vi "Update_STS_ZSpec_Param_SubVI.vi"(4 "ZSpec Param List #5":u16, 5 "Boolean":bool, 6 "STS Param List #5":u16, 7 "reference in":refnum<vi>, 8 "reference 4":refnum<vi>, 9 "reference 3":refnum<vi>, 10 "Experiment 6":T1, 11 "Path in":refnum<vi>) -> (3 "Experiment 5":T1)   [LabVIEW 2014]
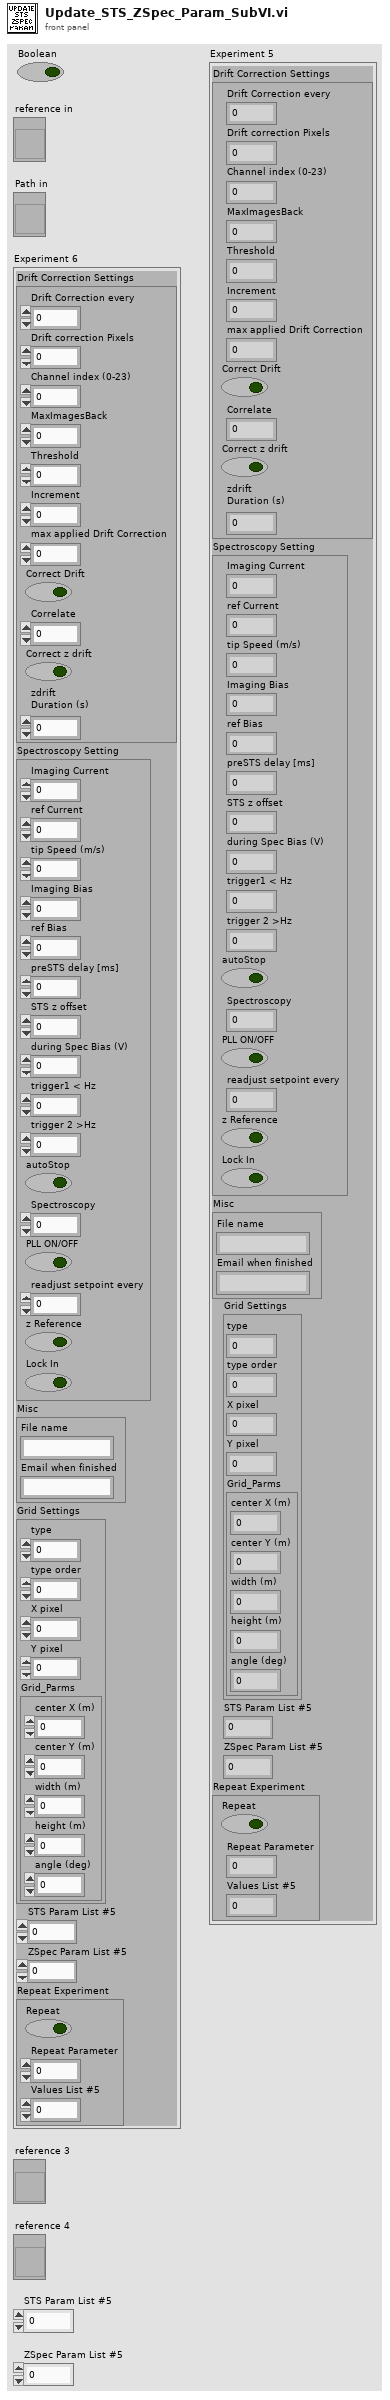
[diagram p1: front panel]
types:
  T1 = cluster{"Drift Correction Settings":cluster{"Drift Correction every":i32, "Drift correction Pixels":i32, "Channel index (0-23)":u8, "MaxImagesBack":i32, "Threshold":i32, "Increment":i32, "max applied Drift Correction":i32, "Correct Drift":bool, "Correlate":u16, "Correct z drift":bool, "zdrift \nDuration (s)":dbl}, "Spectroscopy Setting":cluster{"Imaging Current":dbl, "ref Current":dbl, "tip Speed (m/s)":sgl, "Imaging Bias":dbl, "ref Bias":dbl, "preSTS delay [ms]":u32, "STS z offset":dbl, "during Spec Bias (V)":sgl, "trigger1 < Hz":sgl, "trigger 2 >Hz":sgl, "autoStop":bool, "Spectroscopy":u16, "PLL ON/OFF":bool, "readjust setpoint every ":i32, "z Reference":bool, "Lock In":bool}, "Misc":cluster{"File name":string, "Email when finished":string}, "Grid Settings":cluster{"type":u16, "type order":u16, "X pixel":i32, "Y pixel":i32, "Grid_Parms":cluster{"center X (m)":sgl, "center Y (m)":sgl, "width (m)":sgl, "height (m)":sgl, "angle (deg)":sgl}}, "STS Param List #5 ":u16, "ZSpec Param List #5  ":u16, "Repeat Experiment":cluster{"Repeat":bool, "Repeat Parameter":u16, "Values List #5":i32}}
  T2 = cluster{"Amplitude (mod. signal unit)":sgl, "Lockin on/off status":bool, "Backward sweep":bool, "Number of points":i32, "Channels":string[], "Parameters":string[], "Fixed parameters":string[], "Multiple sweeps configuration":cluster{"Number of Sweeps":i32, "Save all":bool}, "Initialization":cluster{"Z averaging time (s)":sgl, "Initial settling time (s)":sgl}, "Sweep Timing":cluster{"Max. slew rate (V/s)":sgl, "Settling time (s)":sgl, "Integration time (s)":sgl}, "End of Sweep":cluster{"End settling time (s)":sgl, "Z control time (s)":sgl}, "Initial Z-Offset (m)":sgl, "Sweep Distance (m)":sgl, "Channels 2":i32[], "Name":string, "Reset Z":bool, "Record final Z":bool, "Auto Retract Status":bool, "Threshold":sgl, "Auto Retract Signal Index":i32, "Auto Retract Condition":bool}[]
  T3 = cluster{"Amplitude (mod. signal unit)":sgl, "Lockin on/off status":bool, "Backward sweep":bool, "Number of points":i32, "Channels":string[], "Parameters":string[], "Fixed parameters":string[], "Multiple sweeps configuration":cluster{"Number of Sweeps":i32, "Save all":bool}, "Initialization":cluster{"Z averaging time (s)":sgl, "Initial settling time (s)":sgl}, "Sweep Timing":cluster{"Max. slew rate (V/s)":sgl, "Settling time (s)":sgl, "Integration time (s)":sgl}, "End of Sweep":cluster{"End settling time (s)":sgl, "Z control time (s)":sgl}, "Initial Z-Offset (m)":sgl, "Sweep Distance (m)":sgl, "Channels 2":i32[], "Name":string, "Reset Z":bool, "Record final Z":bool, "Auto Retract Status":bool, "Threshold":sgl, "Auto Retract Signal Index":i32, "Auto Retract Condition":bool}
  T4 = cluster{"Amplitude (mod. signal unit)":sgl, "Lockin on/off status":bool, "Advanced options":cluster{"Z-Controller Hold":bool, "Record final Z":bool, "Reset Bias":bool}, "Backward sweep":bool, "Number of points":i32, "Channels":string[], "Parameters":string[], "Fixed parameters":string[], "Multiple sweeps configuration":cluster{"Number of Sweeps":i32, "Save all":bool}, "Initialization":cluster{"Z averaging time (s)":sgl, "Z offset (m)":sgl, "Initial settling time (s)":sgl}, "Sweep Timing":cluster{"Max. slew rate (V/s)":sgl, "Settling time (s)":sgl, "Integration time (s)":sgl}, "End of Sweep":cluster{"End settling time (s)":sgl, "Z control time (s)":sgl}, "Start value (V)":sgl, "End value (V)":sgl, "Channels 2":i32[], "Name":string}[]
  T5 = cluster{"Amplitude (mod. signal unit)":sgl, "Lockin on/off status":bool, "Advanced options":cluster{"Z-Controller Hold":bool, "Record final Z":bool, "Reset Bias":bool}, "Backward sweep":bool, "Number of points":i32, "Channels":string[], "Parameters":string[], "Fixed parameters":string[], "Multiple sweeps configuration":cluster{"Number of Sweeps":i32, "Save all":bool}, "Initialization":cluster{"Z averaging time (s)":sgl, "Z offset (m)":sgl, "Initial settling time (s)":sgl}, "Sweep Timing":cluster{"Max. slew rate (V/s)":sgl, "Settling time (s)":sgl, "Integration time (s)":sgl}, "End of Sweep":cluster{"End settling time (s)":sgl, "Z control time (s)":sgl}, "Start value (V)":sgl, "End value (V)":sgl, "Channels 2":i32[], "Name":string}
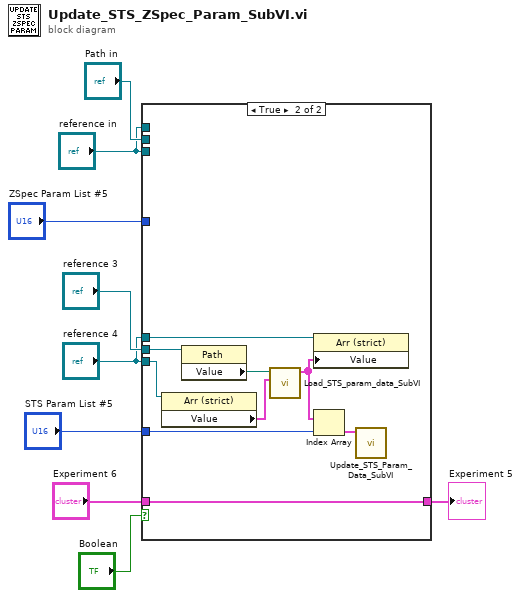
[diagram p0: block diagram]
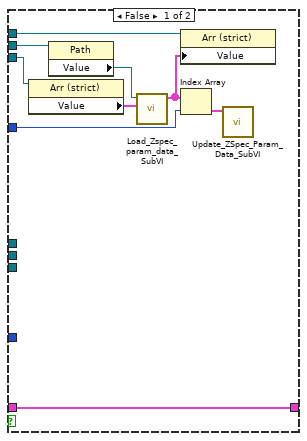
[diagram p2: hidden frame]
diagram:
  n1 = case shown="True" "Boolean" {
    tunnel: "ZSpec Param List #5" -> [w15 _]
    tunnel: "STS Param List #5" -> [_ w25]
    tunnel: "Experiment 6" -> [w18 w27]
    tunnel: [w18 w27] -> w9
    tunnel: "Path in" -> [w12 _]
    tunnel: "reference in" -> [w11 _]
    tunnel: "reference in" -> [w10 _]
    tunnel: "reference 3" -> [_ w21]
    tunnel: "reference 4" -> [_ w20]
    tunnel: "reference 4" -> [_ w19]
    frame False {
      n2 = property class="Arr (strict)"(reference=w10) -> ("Value"=w14:T2)  [unwired: 1 in, 2 out]
      n3 = property class="Path"(reference=w12) -> ("Value"=w13:path)  [unwired: 1 in, 2 out]
      n4 = call "Load_Zspec_param_data_SubVI.vi"("data\n\n 5"=w14, "Zspecparam.txt location"=w13) -> ("data"=w16:T2)  [unwired: 9 in]
      n5 = property class="Arr (strict)"(reference=w11, "Value"=w16) -> ()  [unwired: 1 in, 2 out]
      n6 = Index Array(array=w16, index=w15) -> (element=w17:T3)
      n7 = call "Update_ZSpec_Param_Data_SubVI.vi"("output cluster"=w17) -> ()  [unwired: 11 in]
    }
    frame True {
      n8 = property class="Arr (strict)"(reference=w19) -> ("Value"=w23:T4)  [unwired: 1 in, 2 out]
      n9 = property class="Path"(reference=w21) -> ("Value"=w22:path)  [unwired: 1 in, 2 out]
      n10 = call "Load_STS_param_data_SubVI.vi"("data\n\n in"=w23, "STSparam.txt location"=w22) -> ("data\n\n out"=w24:T4)  [unwired: 9 in]
      n11 = property class="Arr (strict)"(reference=w20, "Value"=w24) -> ()  [unwired: 1 in, 2 out]
      n12 = Index Array(array=w24, index=w25) -> (element=w26:T5)
      n13 = call "Update_STS_Param_Data_SubVI.vi"("STSparameters"=w26) -> ()  [unwired: 11 in]
    }
  }
  "Experiment 5" <- w9
